vi "Parse Blob Service Properties.vi"(11 "Blob service string":string) -> (3 "Blob service properties":T1)   [LabVIEW 2015, in "NI_Azure_Blob.lvlib"]
uses:
  NI_Azure_Blob.lvlib
  Blob Service Properties.ctl
  Logging.ctl
  Retention Policy.ctl
  Metrics.ctl
  Cors Rule.ctl
  XML Parsing/NI_Azure_XML Parsing.lvlib
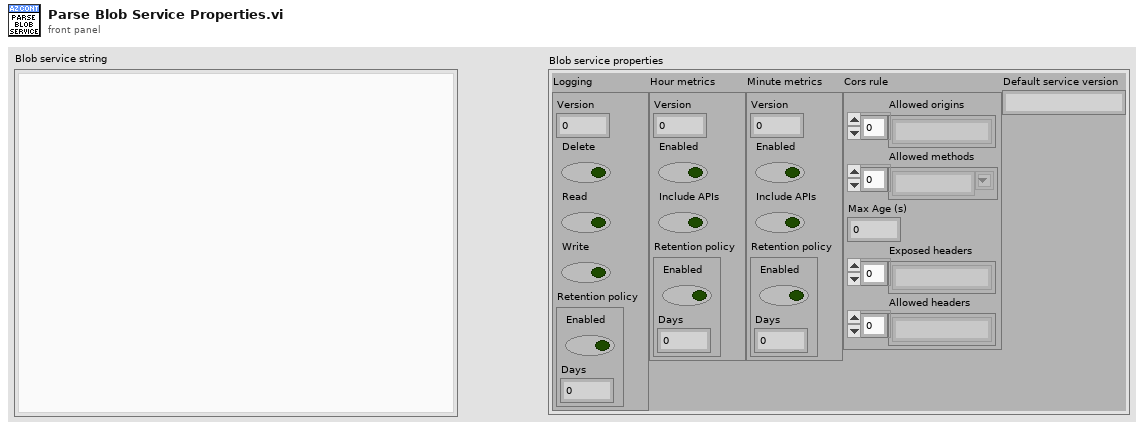
[diagram p1: front panel]
types:
  T1 = typedef "NI_Azure_Blob.lvlib/Blob Service Properties.ctl" = cluster{"Logging":T2, "Hour metrics":T4, "Minute metrics":T4, "Cors rule":T5, "Default service version":string}
  T2 = typedef "NI_Azure_Blob.lvlib/Logging.ctl" = cluster{"Version":dbl, "Delete":bool, "Read":bool, "Write":bool, "Retention policy":T3}
  T3 = typedef "NI_Azure_Blob.lvlib/Retention Policy.ctl" = cluster{"Enabled":bool, "Days":u32}
  T4 = typedef "NI_Azure_Blob.lvlib/Metrics.ctl" = cluster{"Version":dbl, "Enabled":bool, "Include APIs":bool, "Retention policy":T3}
  T5 = typedef "NI_Azure_Blob.lvlib/Cors Rule.ctl" = cluster{"Allowed origins":string[], "Allowed methods":string[], "Max Age (s)":u32, "Exposed headers":string[], "Allowed headers":string[]}
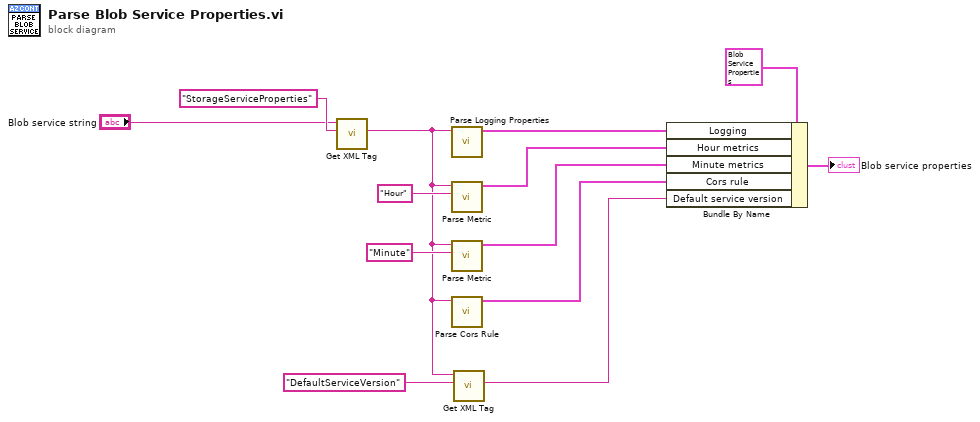
[diagram p0: block diagram]
diagram:
  n1 = call "Get XML Tag.vi"("Tag name"="StorageServiceProperties", "XML String in"="Blob service string") -> ("Tag value"=w4:string)  [unwired: 5 in, 4 out]
  n2 = call "Parse Logging Properties.vi"("String"=w4) -> ("Logging properties"=w10:T2)  [unwired: 10 in]
  n3 = call "Parse Metric.vi"("Metric name"="Hour", "String"=w4) -> ("Metric properties"=w8:T4)  [unwired: 9 in]
  n4 = call "Parse Metric.vi"("Metric name"="Minute", "String"=w4) -> ("Metric properties"=w6:T4)  [unwired: 9 in]
  n5 = call "Parse Cors Rule.vi"("String"=w4) -> ("Cors rule"=w5:T5)  [unwired: 10 in]
  n6 = call "Get XML Tag.vi"("Tag name"="DefaultServiceVersion", "XML String in"=w4) -> ("Tag value"=w2:string)  [unwired: 5 in, 4 out]
  n7 = Bundle By Name(cluster=T1 {"Logging"={"Version"=0.0, "Delete"=FALSE, "Read"=FALSE, "Write"=FALSE, "Retention policy"={"Enabled"=FALSE, "Days"=0}}, "Hour metrics"={"Version"=0.0, "Enabled"=FALSE, "Include APIs"=FALSE, "Retention policy"={"Enabled"=FALSE, "Days"=0}}, "Minute metrics"={"Version"=0.0, "Enabled"=FALSE, "Include APIs"=FALSE, "Retention policy"={"Enabled"=FALSE, "Days"=0}}, "Cors rule"={"Allowed origins"=[], "Allowed methods"=[], "Max Age (s)"=0, "Exposed headers"=[], "Allowed headers"=[]}, "Default service version"=""} ("Blob service properties"), "Logging"=w10, "Hour metrics"=w8, "Minute metrics"=w6, "Cors rule"=w5, "Default service version"=w2) -> (→"Blob service properties":T1)
